vi "1_producer_2_consumersMOD.vi"() -> ()   [LabVIEW 2019]
doc: "Use this template to build a producer/consumer design pattern. Use this template when you need to execute a process, such as data analysis, when a data source, such as a triggered acquisition, produces data at an uneven rate and you need to execute the process when the data becomes available."
panel:
  in  "Enqueue Element":bool
  out "event from consumer loop 2":string
  out "event from consumer loop 1":string
  in  "stop":bool
  # "Run this and notice that only one consumer loop gets each event\n every time you press the \"Enqueue Element\" button.\nI'd like a way that they both get the event."
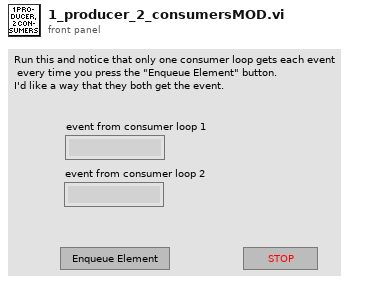
[diagram p1: front panel]
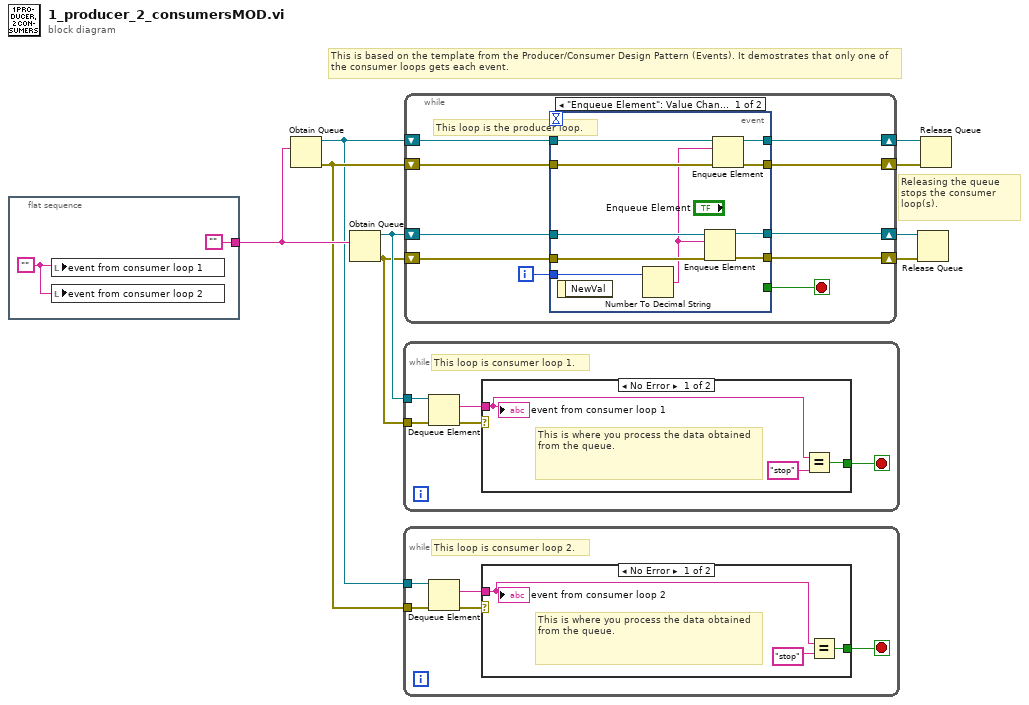
[diagram p0: block diagram]
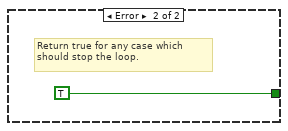
[diagram p2: hidden frame]
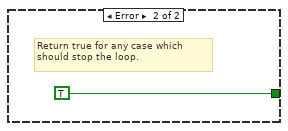
[diagram p3: hidden frame]
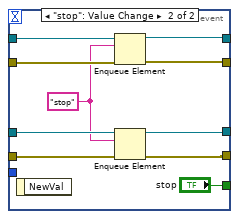
[diagram p4: hidden frame]
diagram:
  # "Releasing the queue stops the consumer loop(s)."
  # "This is based on the template from the Producer/Consumer Design Pattern (Events). It demostrates that only one of the consumer loops gets each event."
  n1 = flat-sequence {
    tunnel: [""] -> w6
    frame #0 {
      w11 = ""
      n2 = local write "event from consumer loop 1"(w11) -> ()
      n3 = local write "event from consumer loop 2"(w11) -> ()
    }
  }
  n4 = Obtain Queue(element data type=w6) -> (queue out=w2:refnum<queue>, error out=w3:errorcluster)  [unwired: 4 in, 1 out]
  n5 = Obtain Queue(element data type=w6) -> (queue out=w7:refnum<queue>, error out=w1:errorcluster)  [unwired: 4 in, 1 out]
  n6 = while {
    tunnel: w7 -> [w16]
    tunnel: w1 -> [w12]
    stop <- w13 stop-if-true
    # "This loop is consumer loop 1."
    n7 = Dequeue Element(queue=w16, error in (no error)=w12) -> (element=w14:string, error out=w15:errorcluster)  [unwired: 1 in, 2 out]
    n8 = case shown="No Error" w15 {
      tunnel: w14 -> [w17 _]
      tunnel: [w19 TRUE] -> w13
      frame No Error {
        # "This is where you process the data obtained from the queue."
        n9 = Equal?(x=w17, y="stop" ("element")) -> (x = y?=w19:bool)
        "event from consumer loop 1" <- w17
      }
      frame Error {
        # "Return true for any case which should stop the loop."
      }
    }
  }
  n10 = while {
    tunnel: w2 -> [w25]
    tunnel: w3 -> [w21]
    stop <- w22 stop-if-true
    # "This loop is consumer loop 2."
    n11 = Dequeue Element(queue=w25, error in (no error)=w21) -> (element=w23:string, error out=w24:errorcluster)  [unwired: 1 in, 2 out]
    n12 = case shown="No Error" w24 {
      tunnel: w23 -> [w26 _]
      tunnel: [w28 TRUE] -> w22
      frame No Error {
        # "This is where you process the data obtained from the queue."
        n13 = Equal?(x=w26, y="stop" ("element")) -> (x = y?=w28:bool)
        "event from consumer loop 2" <- w26
      }
      frame Error {
        # "Return true for any case which should stop the loop."
      }
    }
  }
  n14 = while {
    shift-right: [w36] -> w8
    shift-left: w1 -> [w37]
    shift-right: [w38] -> w9
    shift-left: w7 -> [w39]
    shift-right: [w30] -> w4
    shift-left: w2 -> [w31]
    shift-right: [w32] -> w5
    shift-left: w3 -> [w33]
    i -> [w35]
    stop <- w34 stop-if-true
    # "This loop is the producer loop."
    n15 = event shown="[0] \"Enqueue Element\": Value Change" {
      selector: _ -> [_ _]
      dyn-events: _ -> [_ _]
      timeout: _ -> [_ _]
      tunnel: w39 -> [w49 w52]
      tunnel: [w48 w51] -> w38
      tunnel: w37 -> [w47 w54]
      tunnel: [w46 w53] -> w36
      tunnel: w35 -> [w45 _]
      tunnel: [_ "stop"] -> w34
      tunnel: w33 -> [w44 w58]
      tunnel: [w43 w57] -> w32
      tunnel: w31 -> [w42 w56]
      tunnel: [w41 w55] -> w30
      event "Enqueue Element": Value Change {
        n16 = event-data() -> ()  [unwired: 1 in, 1 out]
        n17 = Number To Decimal String(number=w45) -> (decimal integer string=w40:string)  [unwired: 1 in]
        n18 = Enqueue Element(queue=w49, element=w40, error in (no error)=w47) -> (queue out=w48:refnum<queue>, error out=w46:errorcluster)  [unwired: 1 in, 1 out]
        n19 = Enqueue Element(queue=w42, element=w40, error in (no error)=w44) -> (queue out=w41:refnum<queue>, error out=w43:errorcluster)  [unwired: 1 in, 1 out]
      }
      event "stop": Value Change {
        w50 = "stop" ("element")
        n20 = event-data() -> ()  [unwired: 1 in, 1 out]
        n21 = Enqueue Element(queue=w56, element=w50, error in (no error)=w58) -> (queue out=w55:refnum<queue>, error out=w57:errorcluster)  [unwired: 1 in, 1 out]
        n22 = Enqueue Element(queue=w52, element=w50, error in (no error)=w54) -> (queue out=w51:refnum<queue>, error out=w53:errorcluster)  [unwired: 1 in, 1 out]
      }
    }
  }
  n23 = Release Queue(queue=w9, error in (no error)=w8) -> ()  [unwired: 1 in, 3 out]
  n24 = Release Queue(queue=w4, error in (no error)=w5) -> ()  [unwired: 1 in, 3 out]
